vi "ProyectoFinalArduino.vi"() -> ()   [LabVIEW 2017]
uses:
  Controls/MainControl.ctl
  SubVI/Simulation/Control/SimulationColorTypeEnum.ctl
  SubVI/Simulation/Control/SimulationMainEnum.ctl
  <vilib>/MakerHub/LINX/LMH-LINX.lvlib
  <vilib>/MakerHub/LINX/Private/Device/Type Defs/Pulse Polarity.ctl
  <vilib>/MakerHub/LINX/Private/Device/Device.lvlib
  <vilib>/MakerHub/LINX/Public/Peripherals/Digital/Digital Write N Chans.vi
  <vilib>/MakerHub/LINX/Public/Utilities/Open Serial.vi
panel:
  in  "Mensaje de error":string
  out "VelocidadMotor":dbl
  out "ErrorMsg":string
  out "SimulationErr":bool
  out "Incremento":dbl
  in  "Tab Control 2":enum32{"Page 1", "Page 2"}(tab)
  out "Loading...":u8(slide) scale=0.0..100.0
  in  "Tab Control 3":enum32{"Page 1", "Page 2"}(tab)
  in  "Tab Control":enum32{"Service", "Config"}(tab)
  out "Operario":string
  out "Used Attempts":dbl
  out "TokenColor":T1
  out "TokenVelocity":dbl
  out "Horizontal Pointer Slide":dbl(slide) scale=0.0..20.0
  in  "NewToken":bool
  out "Total De Fichas":dbl
  out "White":dbl
  out "Blue":dbl
  out "Red":dbl
  in  "Stop":bool
  in  "Stop Button":bool
  out "G":dbl
  out "R":dbl
  out "B":dbl
  out "Clear":dbl
  out "Loop Rate (Hz)":u32
  in  "Sensibility":dbl
  out "HistorialDeColoresOutput":string[](array[string])
  in  "Tab Control 4":enum32{"Page 1", "Page 2"}(tab)
  out "hasAccess?":bool
  in  "Grabando?":bool
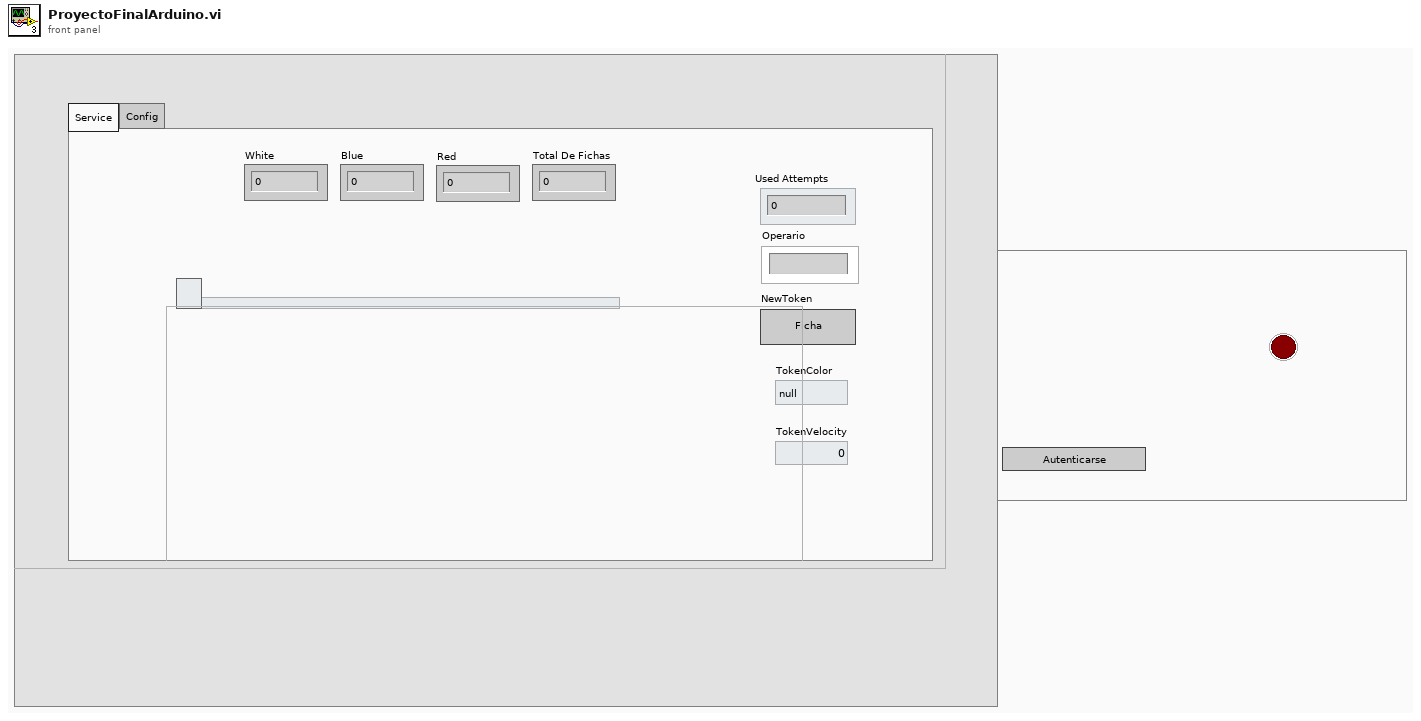
[diagram p1: front panel]
types:
  T1 = typedef "SimulationColorTypeEnum.ctl" = enum16{"null", "White", "Blue", "Red"}
  T2 = typedef "MainControl.ctl" = enum16{"Idle", "VoiceReognition", "Authentication", "Simulation", "Error", "Stop", "Preparation"}
  T3 = typedef "SimulationMainEnum.ctl" = enum16{"idle", "Simulation", "Error", "Stop"}
  T4 = typedef "LMH-LINX.lvlib/LINX Ref.ctl" = cluster{"IO":T5, "Interface":T6, "LINX Device Config":T7}
  T5 = typedef "LMH-LINX.lvlib/Platform.ctl" = enum16{"Remote", "Local"}
  T6 = typedef "LMH-LINX.lvlib/Interface.ctl" = enum16{"Serial", "TCP"}
  T7 = typedef "LMH-LINX.lvlib/Device.lvlib/LINX Device Config.ctl" = cluster{"Interface":T6, "COM Port":refnum<visa-resource-name>, "TCP Configuration":T8, "Device Family":u8, "Device ID":u8, "Device Name":string, "TCP Ref":refnum<k5>, "Channels":T9}
  T8 = typedef "LMH-LINX.lvlib/Device.lvlib/TCP Config.ctl" = cluster{"IP Address":string, "Port":u16}
  T9 = typedef "LMH-LINX.lvlib/Channels.ctl" = cluster{"DI":u8[], "DO":u8[], "AI":u8[], "AO":u8[], "PWM":u8[], "QE":u8[], "UART":u8[], "I2C 2":u8[], "SPI":u8[], "CAN":u8[], "Servo":u8[], "AI Ref (V)":dbl, "AI Resolution (Bits)":u8, "AO Ref (V)":dbl, "AO Resolution (Bits)":u8}
  T10 = typedef "LMH-LINX.lvlib/Device.lvlib/Pulse Polarity.ctl" = enum8{"Active Low", "Active High"}
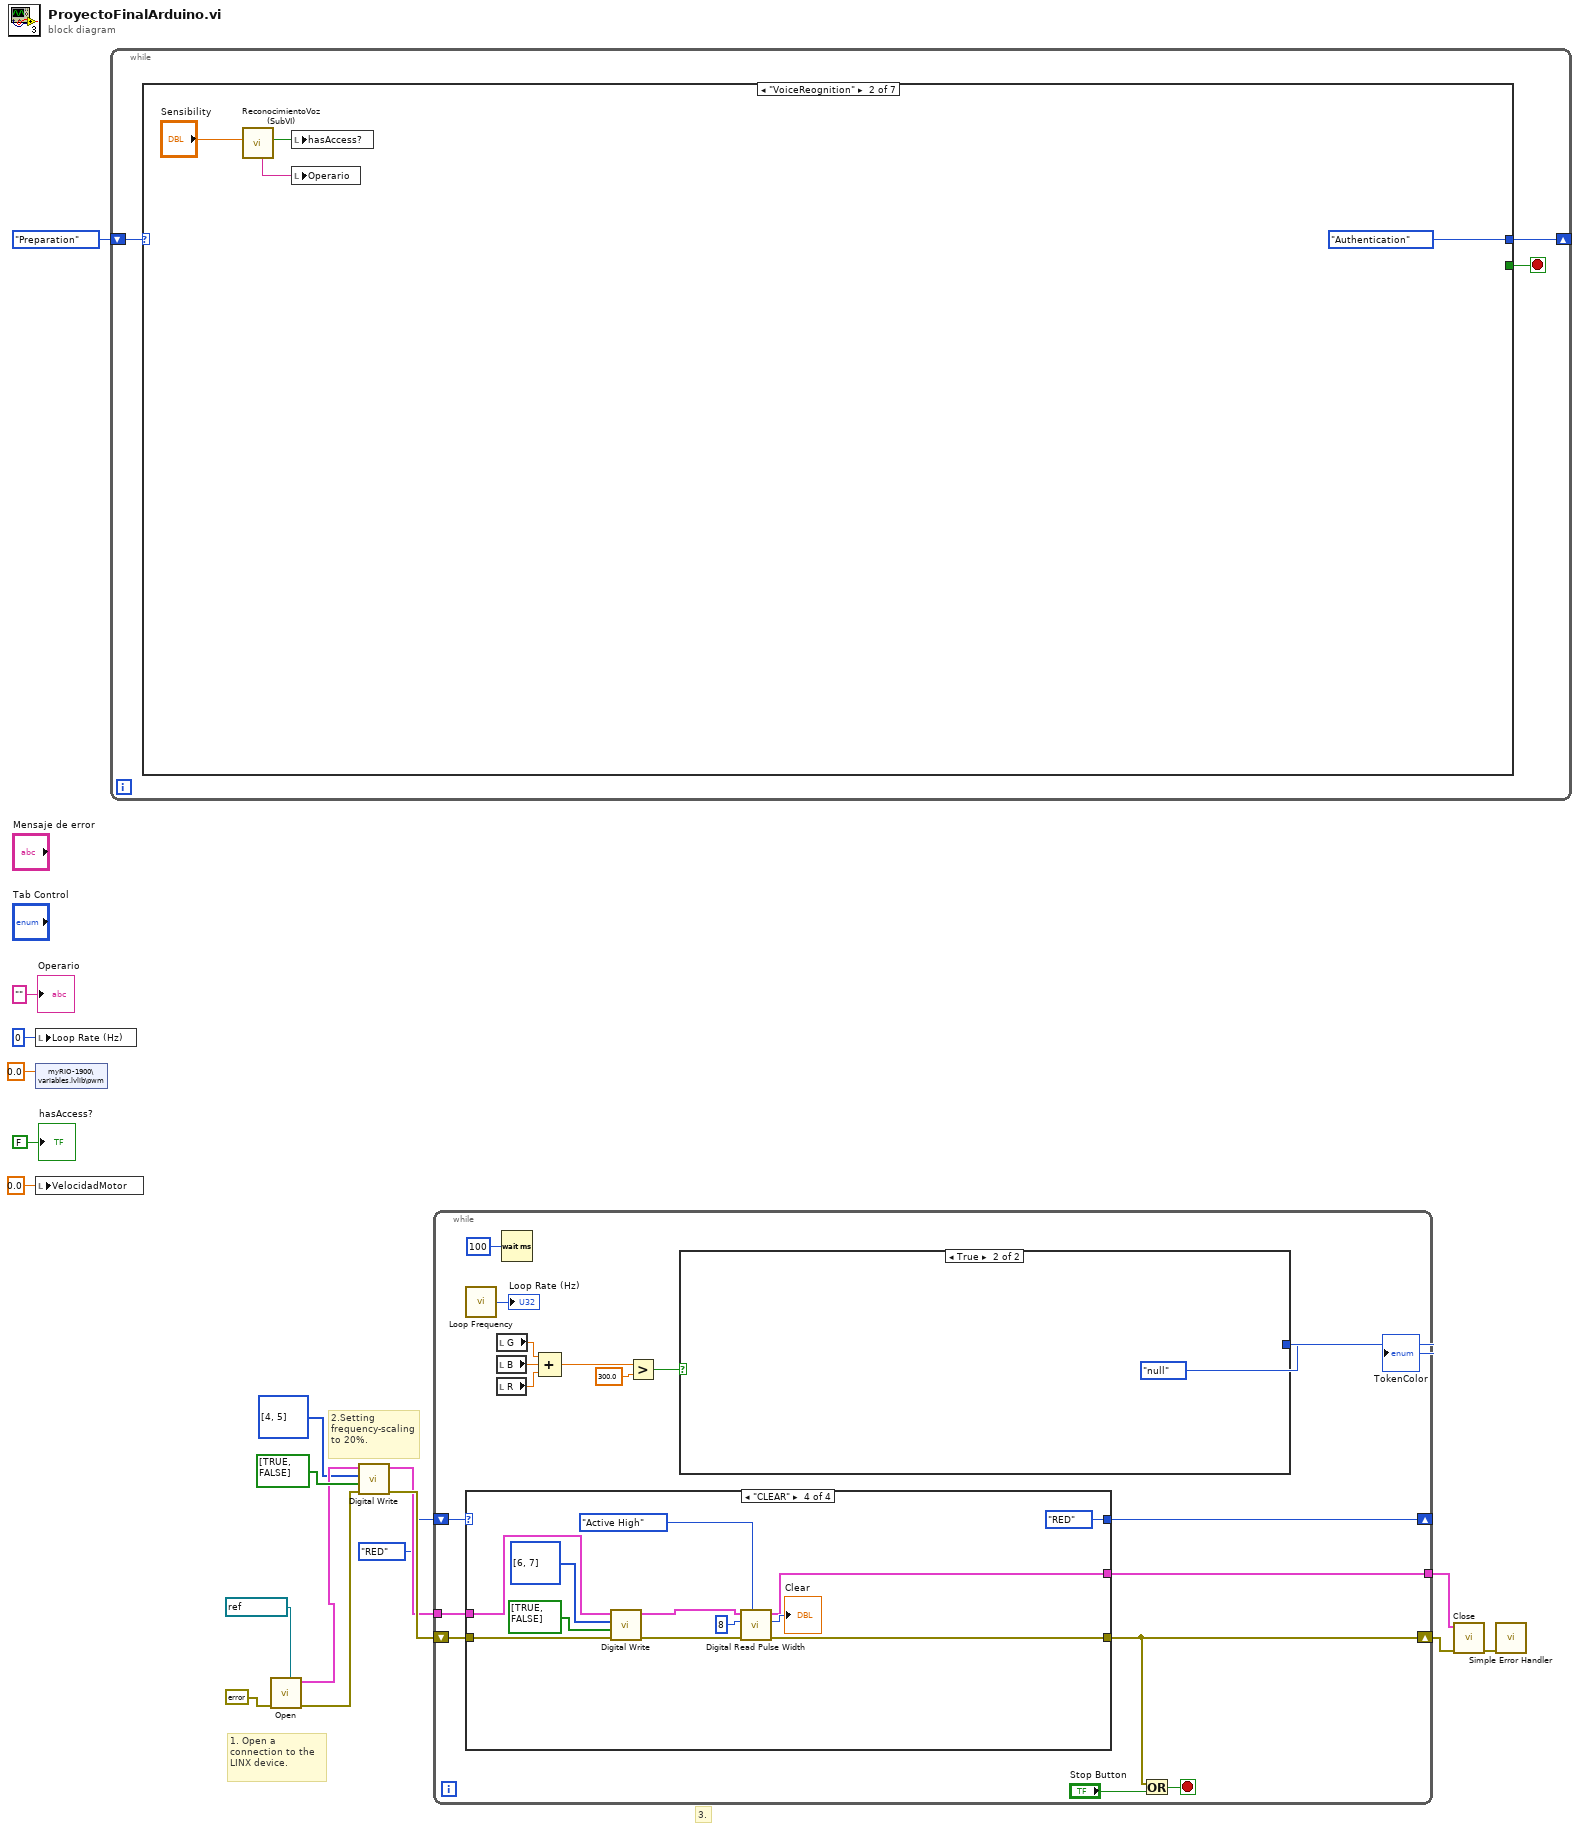
[diagram p0: block diagram]
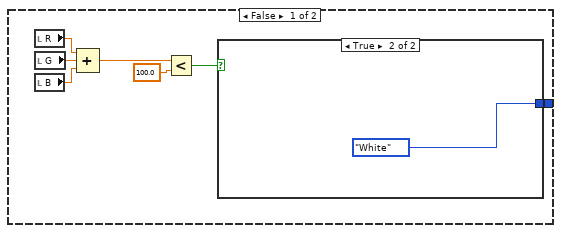
[diagram p2: hidden frame]
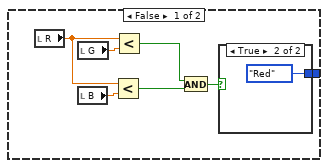
[diagram p3: hidden frame]
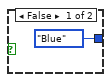
[diagram p4: hidden frame]
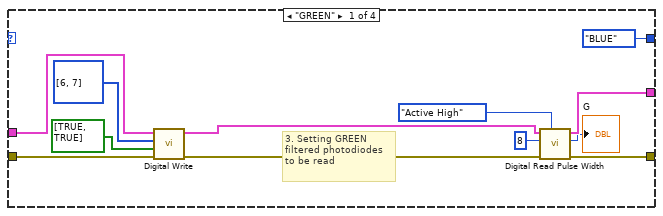
[diagram p5: hidden frame]
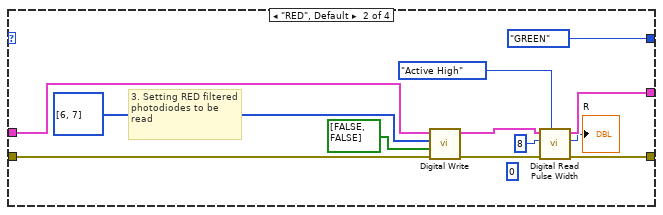
[diagram p6: hidden frame]
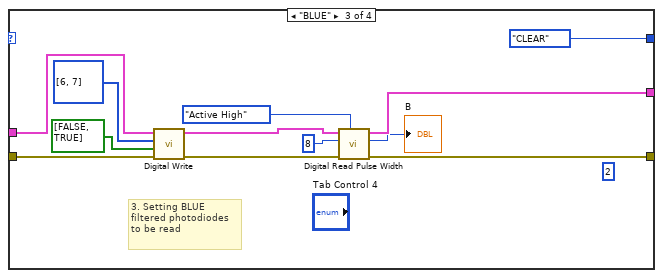
[diagram p7: hidden frame]
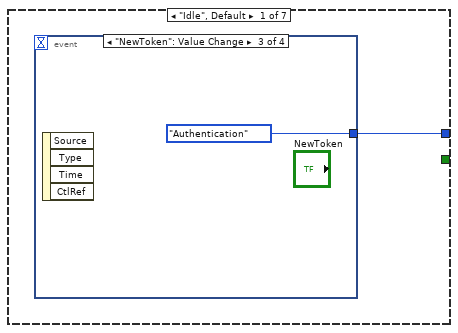
[diagram p8: hidden frame]
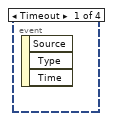
[diagram p9: hidden frame]
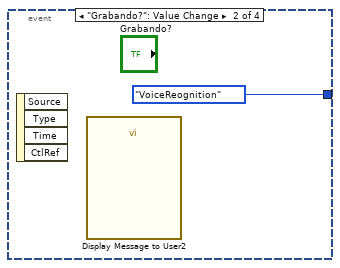
[diagram p10: hidden frame]
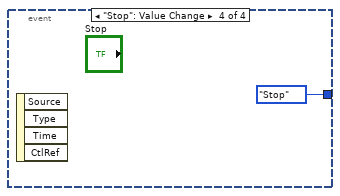
[diagram p11: hidden frame]
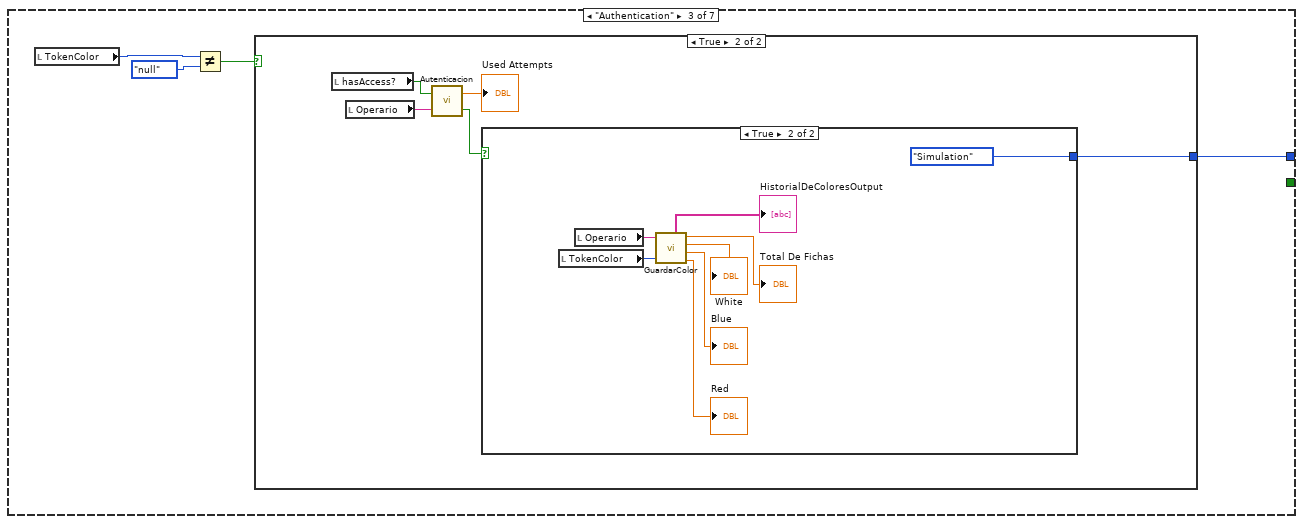
[diagram p12: hidden frame]
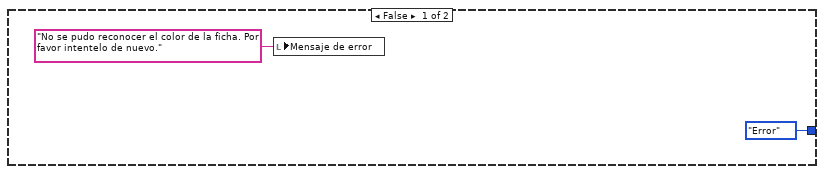
[diagram p13: hidden frame]
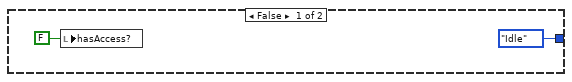
[diagram p14: hidden frame]
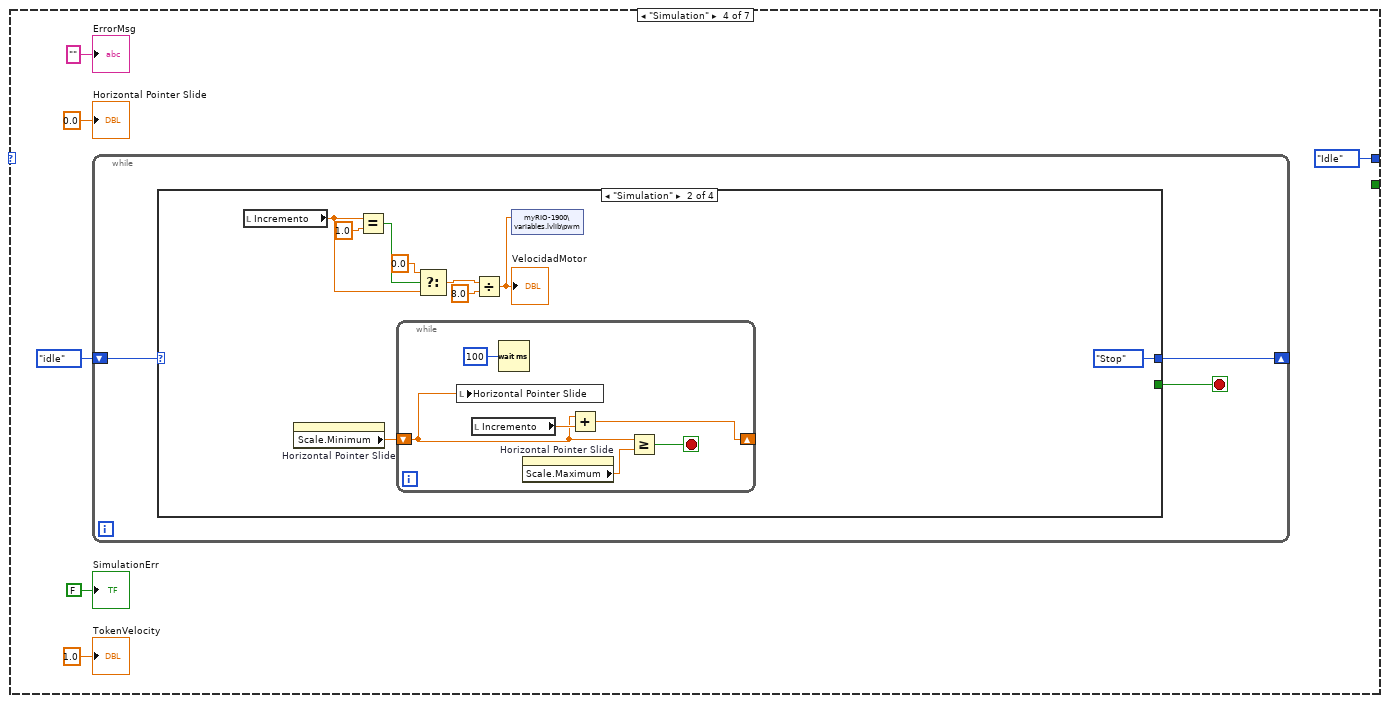
[diagram p15: hidden frame]
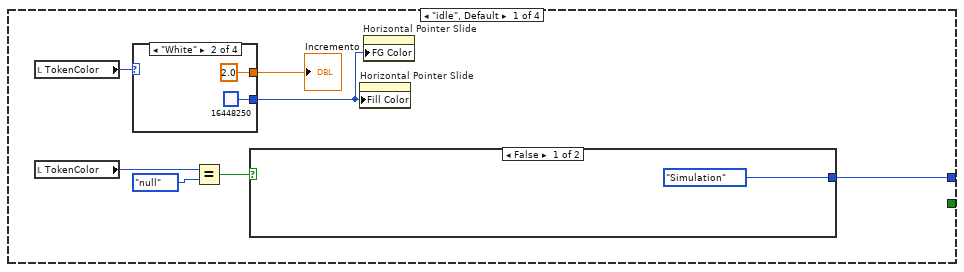
[diagram p16: hidden frame]
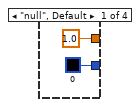
[diagram p17: hidden frame]
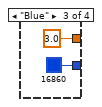
[diagram p18: hidden frame]
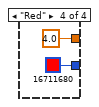
[diagram p19: hidden frame]
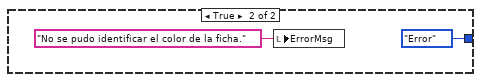
[diagram p20: hidden frame]
diagram:
  # "3."
  # "2.Setting frequency-scaling to 20%."
  # "1. Open a connection to the LINX device."
  n1 = local write "Loop Rate (Hz)"(u32 0 ("Loop Rate (Hz)")) -> ()
  n2 = shared-variable "myRIO-1900\\variables.lvlib\\pwm"(0.0 ("x/y")) -> ()  [unwired: 1 in, 1 out]
  n3 = local write "VelocidadMotor"(0.0 ("x/y")) -> ()
  n4 = while {
    shift-right: [w20] -> _
    shift-left: MainControl."Preparation" -> [w21]
    stop <- w19 stop-if-true
    n5 = case shown="\"VoiceReognition\"" w21 {
      tunnel: [w22 MainControl."Authentication" w33 MainControl."Idle" MainControl."Idle" MainControl."Stop" w112] -> w20
      tunnel: [_ _ _ _ _ TRUE _] -> w19
      frame "Idle", Default {
        n6 = event shown="[2] \"NewToken\": Value Change" {
          selector: _ -> [_ _ _ _]
          dyn-events: _ -> [_ _ _ _]
          timeout: _ -> [_ _ _ _]
          tunnel: [_ MainControl."VoiceReognition" MainControl."Authentication" MainControl."Stop"] -> w22
          event Timeout {
            n7 = event-data() -> ()  [unwired: 1 in, 3 out]
          }
          event "Grabando?": Value Change {
            n8 = event-data() -> ()  [unwired: 1 in, 4 out]
            n9 = call "Display Message to User2"() -> ()  [unwired: 10 in, 2 out]
          }
          event "NewToken": Value Change {
            n10 = event-data() -> ()  [unwired: 1 in, 4 out]
          }
          event "Stop": Value Change {
            n11 = event-data() -> ()  [unwired: 1 in, 4 out]
          }
        }
      }
      frame "VoiceReognition" {
        n12 = call "ReconocimientoVoz (SubVI).vi"("Sensibility"="Sensibility") -> ("hasAccess"=w28:bool, "Name"=w27:string)  [unwired: 7 in, 2 out]
        n13 = local write "hasAccess?"(w28) -> ()
        n14 = local write "Operario"(w27) -> ()
      }
      frame "Authentication" {
        n15 = local read "TokenColor"() -> (w32:T1)
        n16 = Not Equal?(x=w32, y=SimulationColorTypeEnum."null" ("TokenColor")) -> (x != y?=w30:bool)
        n17 = case shown="True" w30 {
          tunnel: [MainControl."Error" w36] -> w33
          frame False {
            n18 = local write "Mensaje de error"("No se pudo reconocer el color de la ficha. Por favor intentelo de nuevo." ("Mensaje de error")) -> ()
          }
          frame True {
            n19 = local read "hasAccess?"() -> (w39:bool)
            n20 = local read "Operario"() -> (w38:string)
            n21 = call "Autenticacion.vi"("Operario"=w38, "TieneAcceso?"=w39) -> ("AccesoPermitido"=w37:bool, "IntentosUsados"=→"Used Attempts":dbl)
            n22 = case shown="True" w37 {
              tunnel: [MainControl."Idle" MainControl."Simulation"] -> w36
              frame False {
                n23 = local write "hasAccess?"(FALSE ("hasAccess?")) -> ()
              }
              frame True {
                n24 = local read "TokenColor"() -> (w48:T1)
                n25 = local read "Operario"() -> (w49:string)
                n26 = call "GuardarColor.vi"("NombreOperario"=w49, "TokenColor"=w48) -> ("HistorialDeColoresOutput"=→"HistorialDeColoresOutput":string[], "Total De Fichas"=→"Total De Fichas":dbl, "White"=→"White":dbl, "Blue"=→"Blue":dbl, "Red"=→"Red":dbl)  [unwired: 4 in]
              }
            }
          }
        }
      }
      frame "Simulation" {
        n27 = while {
          shift-right: [w58] -> _
          shift-left: SimulationMainEnum."idle" -> [w59]
          stop <- w57 stop-if-true
          n28 = case shown="\"Simulation\"" w59 {
            tunnel: [w64 SimulationMainEnum."Stop" SimulationMainEnum."Simulation" SimulationMainEnum."Stop"] -> w58
            tunnel: [_ _ _ TRUE] -> w57
            frame "idle", Default {
              n29 = local read "TokenColor"() -> (w63:T1)
              n30 = local read "TokenColor"() -> (w61:T1)
              n31 = case shown="\"White\"" w63 {
                tunnel: [u32 0 ("Color Box") u32 16448250 ("Color Box") u32 16860 ("Color Box") u32 16711680 ("Color Box")] -> w60
                tunnel: [1.0 ("Incremento") 2.0 ("Incremento") 3.0 ("Incremento") 4.0 ("Incremento")] -> w62
                frame "null", Default {
                }
                frame "White" {
                }
                frame "Blue" {
                }
                frame "Red" {
                }
              }
              "Incremento" <- w62
              n32 = Equal?(x=w61, y=SimulationColorTypeEnum."null") -> (x = y?=w65:bool)
              n33 = case shown="False" w65 {
                tunnel: [SimulationMainEnum."Simulation" SimulationMainEnum."Error"] -> w64
                frame False {
                }
                frame True {
                  n34 = local write "ErrorMsg"("No se pudo identificar el color de la ficha." ("ErrorMsg")) -> ()
                }
              }
              n35 = property on="Horizontal Pointer Slide" class="Slide (strict)"("Fill Color"=w60) -> ()  [unwired: 2 in, 2 out]
              n36 = property on="Horizontal Pointer Slide" class="Slide (strict)"("FG Color"=w60) -> ()  [unwired: 2 in, 2 out]
            }
            frame "Simulation" {
              n37 = local read "Incremento"() -> (w80:dbl)
              n38 = property on="Horizontal Pointer Slide" class="Slide (strict)"() -> ("Scale.Minimum"=w85:dbl)  [unwired: 2 in, 2 out]
              n39 = Equal?(x=w80, y=1.0) -> (x = y?=w82:bool)
              n40 = while {
                shift-right: [w91] -> _
                shift-left: w85 -> [w90]
                stop <- w89 stop-if-true
                n41 = local write "Horizontal Pointer Slide"(w90) -> ()
                n42 = local read "Incremento"() -> (w92:dbl)
                n43 = Wait (ms)(milliseconds to wait=u32 100) -> ()  [unwired: 1 out]
                n44 = property on="Horizontal Pointer Slide" class="Slide (strict)"() -> ("Scale.Maximum"=w88:dbl)  [unwired: 2 in, 2 out]
                n45 = Add(x=w90, y=w92) -> (x+y=w91:dbl)
                n46 = Greater Or Equal?(x=w90, y=w88) -> (x >= y?=w89:bool)
              }
              n47 = Select(t=0.0, s=w82, f=w80) -> (s? t:f=w79:dbl)
              n48 = Divide(x=w79, y=8.0) -> (x/y=w78:dbl)
              "VelocidadMotor" <- w78
              n49 = shared-variable "myRIO-1900\\variables.lvlib\\pwm"(w78) -> ()  [unwired: 1 in, 1 out]
            }
            frame "Error" {
              n50 = local write "SimulationErr"(TRUE ("Boolean")) -> ()
              n51 = local read "ErrorMsg"() -> (w93:string)
              n52 = call "Display Message to User"("Message"=w93) -> ()  [unwired: 9 in, 2 out]
            }
            frame "Stop" {
              w96 = 0.0 ("Horizontal Pointer Slide")
              n53 = local write "Horizontal Pointer Slide"(w96) -> ()
              n54 = local write "VelocidadMotor"(w96) -> ()
              n55 = shared-variable "myRIO-1900\\variables.lvlib\\pwm"(w96) -> ()  [unwired: 1 in, 1 out]
            }
          }
        }
        "TokenVelocity" <- 1.0 ("VelocidadFicha")
        "SimulationErr" <- FALSE ("Boolean")
        "Horizontal Pointer Slide" <- 0.0 ("Horizontal Pointer Slide")
        "ErrorMsg" <- "" ("ErrorMsg")
      }
      frame "Error" {
        n56 = local read "Mensaje de error"() -> (w99:string)
        n57 = call "Display Message to User3"("Message"=w99) -> ()  [unwired: 9 in, 2 out]
      }
      frame "Stop" {
      }
      frame "Preparation" {
        n58 = property on="Tab Control 2" class="TabCtl (strict)"("Visible"=TRUE) -> ()  [unwired: 2 in, 2 out]
        n59 = property on="Loading..." class="Slide (strict)"("Visible"=TRUE) -> ()  [unwired: 2 in, 2 out]
        n60 = property on="Tab Control" class="TabCtl (strict)"("Visible"=FALSE ("Tabs Visible?")) -> ()  [unwired: 2 in, 2 out]
        n61 = property on="Loading..." class="Slide (strict)"() -> ("Scale.Minimum"=w105:dbl)  [unwired: 2 in, 2 out]
        n62 = while {
          shift-right: [w117] -> _
          shift-left: w105 -> [w116]
          stop <- w114 stop-if-true
          n63 = Wait (ms)(milliseconds to wait=u32 10) -> ()  [unwired: 1 out]
          n64 = property on="Loading..." class="Slide (strict)"() -> ("Scale.Maximum"=w115:dbl)  [unwired: 2 in, 2 out]
          n65 = Greater Or Equal?(x=w116, y=w115) -> (x >= y?=w114:bool)
          n66 = Increment(x=w116) -> (x+1=w117:dbl)
          "Loading..." <- w116
        }
        n67 = local read "Loop Rate (Hz)"() -> (w111:u32)
        n68 = Not Equal To 0?(x=w111) -> (x != 0?=w108:bool)
        n69 = Less Or Equal?(x=w111, y=u32 100) -> (x <= y?=w109:bool)
        n70 = And(x=w109, y=w108) -> (x .and. y?=w107:bool)
        n71 = case shown="True" w107 {
          tunnel: [MainControl."Preparation" MainControl."Idle"] -> w112
          frame False {
          }
          frame True {
            n72 = property on="Loading..." class="Slide (strict)"("Visible"=FALSE) -> ()  [unwired: 2 in, 2 out]
            n73 = property on="Tab Control" class="TabCtl (strict)"("Visible"=TRUE ("Tabs Visible?")) -> ()  [unwired: 2 in, 2 out]
            n74 = property on="Tab Control 2" class="TabCtl (strict)"("Visible"=FALSE) -> ()  [unwired: 2 in, 2 out]
          }
        }
      }
    }
  }
  n75 = call-poly <vilib>:"Open.vi"("Error In"=errorcluster {"status"=FALSE, "code"=0, "source"=""}, "Serial Port"=refnum<visa-resource-name> "COM7") -> ("Error Out"=w8:errorcluster, "LINX Resource"=w6:T4)  [unwired: 7 in, 1 out]
  n76 = call-poly <vilib>:"Digital Write.vi"("Error In"=w8, "Values"=bool[] [TRUE, FALSE], "DO Channels"=i32[] [4, 5], "LINX Resource"=w6) -> ("Error Out"=w12:errorcluster, "LINX Resource"=w11:T4)  [unwired: 6 in]
  n77 = while {
    shift-right: [w125] -> w3
    shift-left: w12 -> [w136]
    tunnel: w11 -> [w135]
    tunnel: [w126] -> w4
    shift-right: [w132] -> _
    shift-left: enum16{"RED", "GREEN", "BLUE", "CLEAR"}."RED" -> [w134]
    stop <- w139 stop-if-true
    n78 = call <vilib>:"Loop Frequency.vi"() -> ("Loop Rate (Hz)"=→"Loop Rate (Hz)":u32)
    n79 = case shown="\"CLEAR\"" w134 {
      tunnel: w136 -> [w166 w178 w189 w204]
      tunnel: w135 -> [w169 w176 w190 w205]
      tunnel: [w167 w181 w193 w199] -> w126
      tunnel: [w162 w180 w191 w197] -> w125
      tunnel: [enum16{"RED", "GREEN", "BLUE", "CLEAR"}."BLUE" enum16{"RED", "GREEN", "BLUE", "CLEAR"}."GREEN" enum16{"RED", "GREEN", "BLUE", "CLEAR"}."CLEAR" enum16{"RED", "GREEN", "BLUE", "CLEAR"}."RED"] -> w132
      frame "GREEN" {
        # "3. Setting GREEN filtered photodiodes to be read"
        n80 = call-poly <vilib>:"Digital Write.vi"("Error In"=w166, "Values"=bool[] [TRUE, TRUE], "DO Channels"=i32[] [6, 7], "LINX Resource"=w169) -> ("Error Out"=w165:errorcluster, "LINX Resource"=w168:T4)  [unwired: 6 in]
        n81 = call <vilib>:"Digital Read Pulse Width.vi"("Incoming Pulse Polarity (Active High)"=Pulse_Polarity."Active High", "Error In"=w165, "DI Channel"=8, "LINX Resource"=w168) -> ("Error Out"=w162:errorcluster, "Pulse Width (uS)"=→"G":u32, "LINX Resource"=w167:T4)  [unwired: 5 in]
      }
      frame "RED", Default {
        (unwired) 0 ("index")
        # "3. Setting RED filtered photodiodes to be read"
        n82 = call-poly <vilib>:"Digital Write.vi"("Error In"=w178, "Values"=bool[] [FALSE, FALSE], "DO Channels"=i32[] [6, 7], "LINX Resource"=w176) -> ("Error Out"=w177:errorcluster, "LINX Resource"=w175:T4)  [unwired: 6 in]
        n83 = call <vilib>:"Digital Read Pulse Width.vi"("Incoming Pulse Polarity (Active High)"=Pulse_Polarity."Active High", "Error In"=w177, "DI Channel"=8, "LINX Resource"=w175) -> ("Error Out"=w180:errorcluster, "Pulse Width (uS)"=→"R":u32, "LINX Resource"=w181:T4)  [unwired: 5 in]
      }
      frame "BLUE" {
        (unwired) 2 ("index")
        # "3. Setting BLUE filtered photodiodes to be read"
        n84 = call-poly <vilib>:"Digital Write.vi"("Error In"=w189, "Values"=bool[] [FALSE, TRUE], "DO Channels"=i32[] [6, 7], "LINX Resource"=w190) -> ("Error Out"=w187:errorcluster, "LINX Resource"=w188:T4)  [unwired: 6 in]
        n85 = call <vilib>:"Digital Read Pulse Width.vi"("Incoming Pulse Polarity (Active High)"=Pulse_Polarity."Active High", "Error In"=w187, "DI Channel"=8, "LINX Resource"=w188) -> ("Error Out"=w191:errorcluster, "Pulse Width (uS)"=→"B":u32, "LINX Resource"=w193:T4)  [unwired: 5 in]
      }
      frame "CLEAR" {
        n86 = call-poly <vilib>:"Digital Write.vi"("Error In"=w204, "Values"=bool[] [TRUE, FALSE], "DO Channels"=i32[] [6, 7], "LINX Resource"=w205) -> ("Error Out"=w198:errorcluster, "LINX Resource"=w201:T4)  [unwired: 6 in]
        n87 = call <vilib>:"Digital Read Pulse Width.vi"("Incoming Pulse Polarity (Active High)"=Pulse_Polarity."Active High", "Error In"=w198, "DI Channel"=8, "LINX Resource"=w201) -> ("Error Out"=w197:errorcluster, "Pulse Width (uS)"=→"Clear":u32, "LINX Resource"=w199:T4)  [unwired: 5 in]
      }
    }
    n88 = local read "G"() -> (w131:dbl)
    n89 = local read "B"() -> (w128:dbl)
    n90 = local read "R"() -> (w127:dbl)
    n91 = Wait (ms)(milliseconds to wait=u32 100) -> ()  [unwired: 1 out]
    n92 = Compound Arithmetic op=ADD(w131, w128, w127) -> (w130:dbl)
    n93 = Greater?(x=w130, y=300.0) -> (0:w124:bool)
    n94 = case shown="True" w124 {
      tunnel: [w140 SimulationColorTypeEnum."null" ("TokenColor")] -> w123
      frame False {
        n95 = local read "R"() -> (w146:dbl)
        n96 = local read "G"() -> (w145:dbl)
        n97 = local read "B"() -> (w144:dbl)
        n98 = Compound Arithmetic op=ADD(w146, w145, w144) -> (w142:dbl)
        n99 = Less?(x=w142, y=100.0) -> (x < y?=w141:bool)
        n100 = case shown="True" w141 {
          tunnel: [w147 SimulationColorTypeEnum."White" ("TokenColor")] -> w140
          frame False {
            n101 = local read "R"() -> (w151:dbl)
            n102 = local read "G"() -> (w152:dbl)
            n103 = local read "B"() -> (w153:dbl)
            n104 = Less?(x=w151, y=w153) -> (x < y?=w150:bool)
            n105 = Less?(x=w151, y=w152) -> (x < y?=w149:bool)
            n106 = And(x=w149, y=w150) -> (x .and. y?=w148:bool)
            n107 = case shown="True" w148 {
              tunnel: [SimulationColorTypeEnum."Blue" ("TokenColor") SimulationColorTypeEnum."Red" ("TokenColor")] -> w147
              frame False {
              }
              frame True {
              }
            }
          }
          frame True {
          }
        }
      }
      frame True {
      }
    }
    "TokenColor" <- w123
    n108 = Or(x=w125, y="Stop Button") -> (x .or. y?=w139:bool)
  }
  n109 = call <vilib>:"Close.vi"("Error In"=w3, "LINX Resource"=w4) -> ("Error Out"=w1:errorcluster)  [unwired: 9 in]
  n110 = call <vilib>:"Simple Error Handler.vi"("error in (no error)"=w1) -> ()  [unwired: 4 in, 5 out]
  "Operario" <- "" ("Operario")
  "hasAccess?" <- FALSE ("hasAccess?")
